vi "PlugIn Solenoid.vi"(6 "String Value":string, 10 "Channel":i32) -> ()   [LabVIEW 2019]
uses:
  Solenoid Update Ops.ctl
panel:
  in  "Menu":T1=enum."set init"
  # "Don't place this VI anywhere\nin your API code. It needs to\nbe a dynamically loaded\nwrapper of the main global"
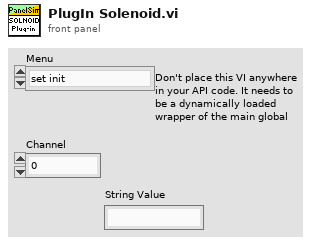
[diagram p1: front panel]
types:
  T1 = typedef "Solenoid Update Ops.ctl" = enum16{"get", "delete", "JSON update", "set  name", "transmit initial", "reset", "set init", "set output"}
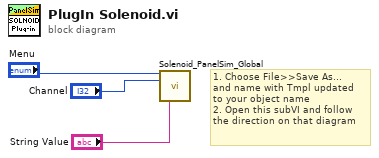
[diagram p0: block diagram]
diagram:
  # "1. Choose File>>Save As...\nand name with Tmpl updated\nto your object name\n2. Open this subVI and follow\nthe direction on that diagram"
  n1 = call "Solenoid_PanelSim_Global.vi"("Menu"="Menu", "Channel"="Channel", "String Value"="String Value") -> ()  [unwired: 11 in, 2 out]
